vi "TiMicSDK.vi"() -> ()   [LabVIEW 2011]
uses:
  TILLPhotonics/DevID.ctl
panel:
  out "Value":string
  out "error out":errorcluster
  out "command":string
  # "version without z"
  # "*.z=\"1..\"\n*.x=\"...\"\n*.y=\"...\"\n*.f1=\"..\"\n*.turret=\"...\"\njeweils .set werte"
  # "stage.x.set=\"update\" for read"
  # "remember state! arrival time? not to sent new command before arrival!"
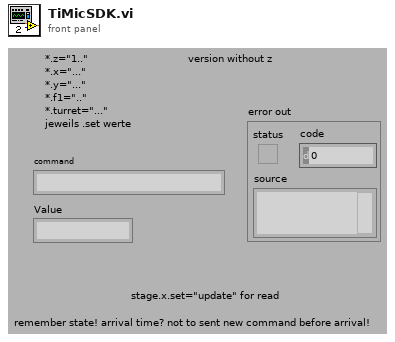
[diagram p1: front panel]
types:
  T1 = enum16{"None/#Datasets", "Clear", "TagValueOf#", "AddValues", "ReadValue", "ChangeValue", "Get all"}
  T2 = cluster{"default value 2":dbl, "default value 1":dbl}
  T3 = typedef "DevID.ctl" = i32
  T4 = enum16{"no error", "missing axis", "missing Z axis", "missing Filter", "iMic not initialized", "no property", "wrong handle", "protocol not finished", "user parameter to long (>32 bits)", "no user parameter handle", "failed to open comport", "failed to initialize"}
  T5 = cluster{bool, "output param":enum16{"no error", "missing axis", "missing Z axis", "missing Filter", "iMic not initialized", "no property", "wrong handle", "protocol not finished", "user parameter to long (>32 bits)", "no user parameter handle", "failed to open comport", "failed to initialize"}, string}
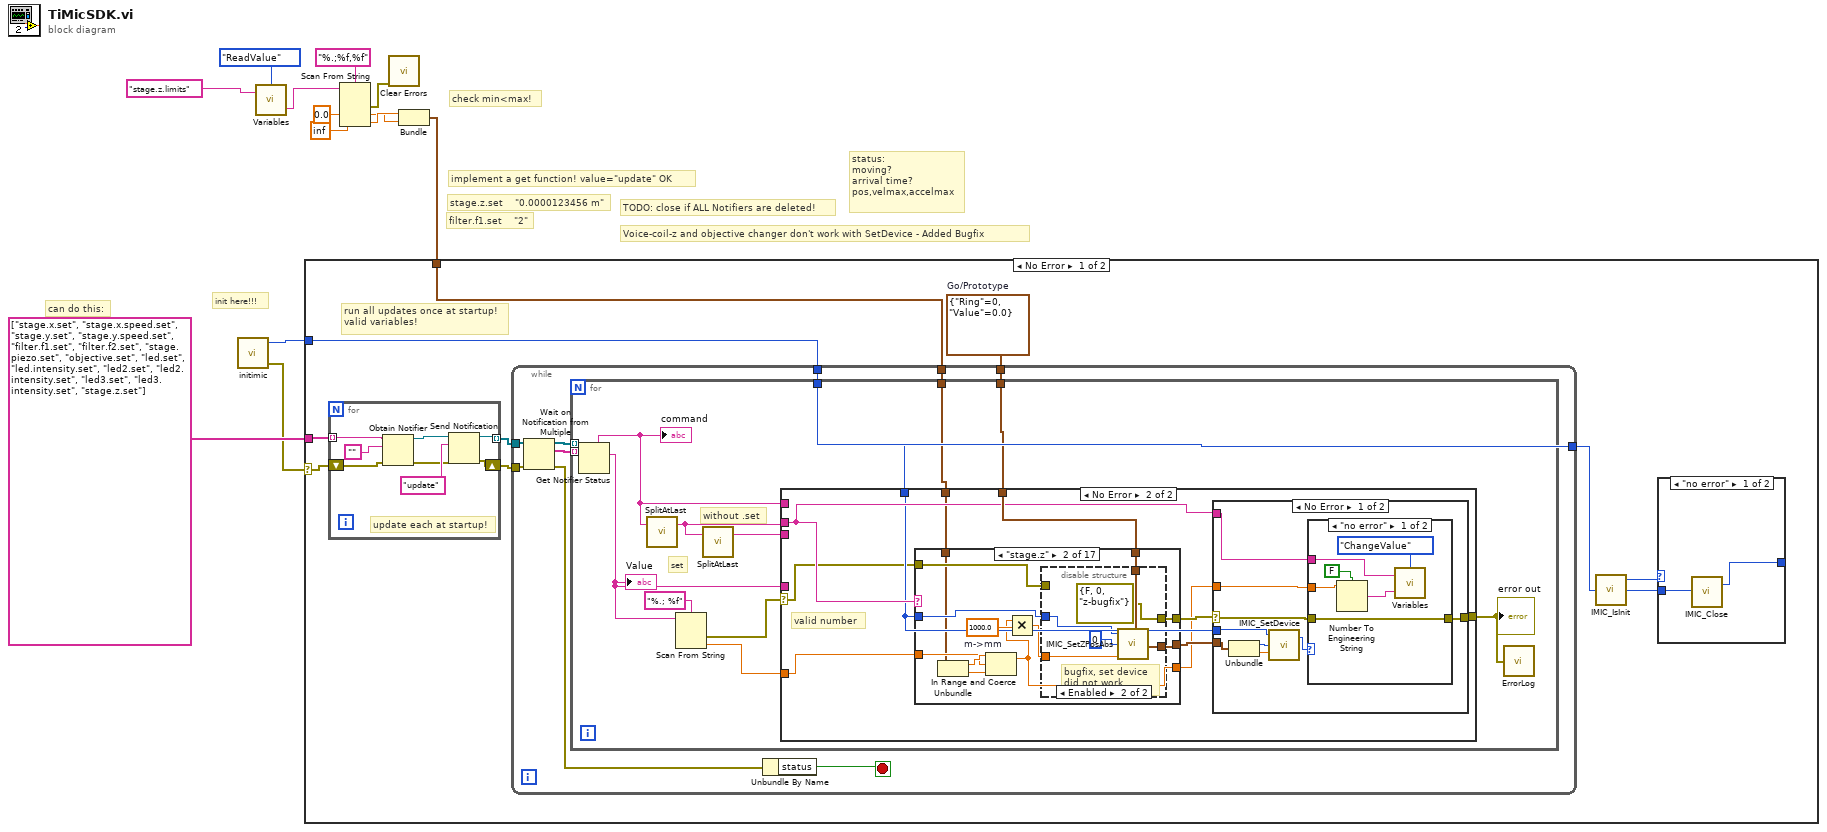
[diagram p0: block diagram]
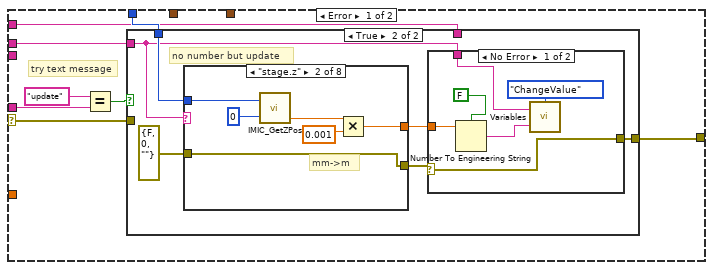
[diagram p3: hidden frame]
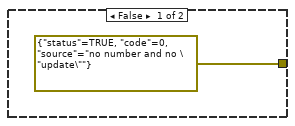
[diagram p4: hidden frame]
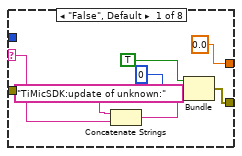
[diagram p6: hidden frame]
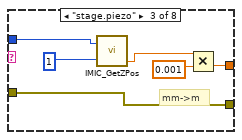
[diagram p7: hidden frame]
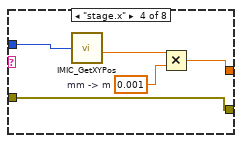
[diagram p8: hidden frame]
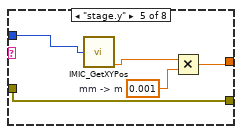
[diagram p9: hidden frame]
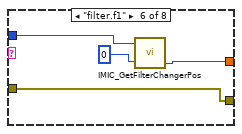
[diagram p10: hidden frame]
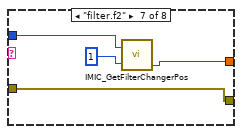
[diagram p11: hidden frame]
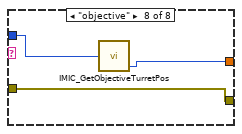
[diagram p12: hidden frame]
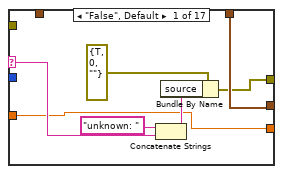
[diagram p13: hidden frame]
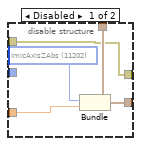
[diagram p14: hidden frame]
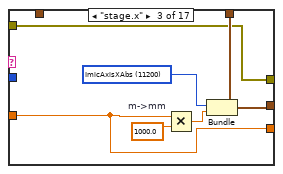
[diagram p15: hidden frame]
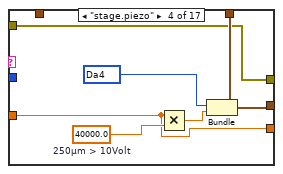
[diagram p16: hidden frame]
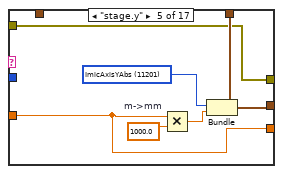
[diagram p17: hidden frame]
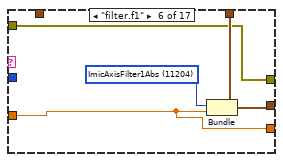
[diagram p18: hidden frame]
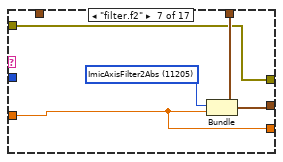
[diagram p19: hidden frame]
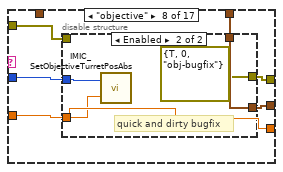
[diagram p20: hidden frame]
diagram:
  # "check min<max!"
  # "can do this:"
  # "Voice-coil-z and objective changer don't work with SetDevice - Added Bugfix"
  # "filter.f1.set    \"2\""
  # "status:\nmoving?\narrival time?\npos,velmax,accelmax"
  # "implement a get function! value=\"update\" OK"
  # "TODO: close if ALL Notifiers are deleted!"
  # "init here!!!"
  # "stage.z.set    \"0.0000123456 m\""
  n1 = call "initimic.vi"() -> ("handle"=w13:u64, "error out"=w11:errorcluster)  [unwired: 3 out]
  n2 = call "Variables.vi"("Tag in"="stage.z.limits", "Command"=T1."ReadValue") -> ("value out"=w8:string)  [unwired: 1 in, 2 out]
  n3 = Scan From String(format string="%.;%f,%f", input string=w8, default 1=0.0 ("default value 1"), default 2=inf ("default value 2")) -> (error out=w2:errorcluster, output 1=w3:dbl, output 2=w4:dbl)  [unwired: 2 in, 2 out]
  n4 = call <vilib>:"Clear Errors.vi"("error in (no error)"=w2) -> ()  [unwired: 7 out]
  n5 = Bundle("default value 2"=w4, "default value 1"=w3) -> (w1:T2)  [unwired: 1 out]
  n6 = case shown="No Error" w11 {
    selector: w11 -> [w15 _]
    tunnel: w13 -> [w23 _]
    tunnel: string[] ["stage.x.set", "stage.x.speed.set", "stage.y.set", "stage.y.speed.set", "filter.f1.set", "filter.f2.set", "stage.piezo.set", "objective.set", "led.set", "led.intensity.set", "led2.set", "led2.intensity.set", "led3.set", "led3.intensity.set", "stage.z.set"] -> [w18 _]
    tunnel: w1 -> [w14 _]
    frame No Error {
      w19 = cluster{"Ring":T3, "Value":dbl} {"Ring"=0, "Value"=0.0}  # Go/Prototype
      # "run all updates once at startup!\nvalid variables!"
      n7 = for {
        tunnel: w18 -> [w31] mode=indexing
        tunnel: [w25] -> w17 mode=indexing
        shift-right: [w24] -> w16
        shift-left: w15 -> [w29]
        # "update each at startup!"
        n8 = Obtain Notifier(name (unnamed)=w31, notification data type="", error in (no error)=w29) -> (notifier out=w27:refnum<notifier>, error out=w26:errorcluster)  [unwired: 1 in, 1 out]
        n9 = Send Notification(notification="update" ("Meldung"), notifier=w27, error in (no error)=w26) -> (notifier out=w25:refnum<notifier>, error out=w24:errorcluster)
      }
      n10 = while {
        tunnel: w17 -> [w38]
        tunnel: w23 -> [w42]
        tunnel: w16 -> [w40]
        tunnel: [w42] -> w21
        tunnel: w19 -> [w41]
        tunnel: w14 -> [w35]
        stop <- w43 stop-if-true
        n11 = Wait on Notification from Multiple(0:w38, 3:w40) -> (8:w37:refnum<notifier>[], 9:w36:string[], 11:w39:errorcluster)  [unwired: 3 out]
        n12 = for {
          tunnel: w42 -> [w55]
          tunnel: w41 -> [w54]
          tunnel: w37 -> [w53] mode=indexing
          tunnel: w36 -> [_] mode=indexing
          tunnel: w35 -> [w44]
          # "without .set"
          # "set"
          n13 = Get Notifier Status(notifier=w53) -> (notifier name=w52:string, current notification=w46:string)  [unwired: 1 in, 3 out]
          "command" <- w52
          "Value" <- w46
          n14 = call "SplitAtLast.vi"("In-String"=w52) -> ("Front (default)"=w51:string)  [unwired: 1 in, 1 out]
          n15 = Scan From String(format string="%.; %f", input string=w46) -> (error out=w47:errorcluster, output 1=w48:dbl)  [unwired: 2 in, 3 out]
          n16 = call "SplitAtLast.vi"("In-String"=w51) -> ("Front (default)"=w50:string)  [unwired: 1 in, 1 out]
          n17 = case shown="No Error" w47 {
            selector: w47 -> [w61 w119]
            tunnel: [w62 w127] -> w45
            tunnel: w55 -> [w63 w122]
            tunnel: w51 -> [w56 w123]
            tunnel: w52 -> [w60 _]
            tunnel: w54 -> [_ w126]
            tunnel: w50 -> [_ _]
            tunnel: w48 -> [_ w121]
            tunnel: w46 -> [w59 _]
            tunnel: w44 -> [_ w118]
            frame Error {
              # "try text message"
              n18 = Equal?(x="update", y=w59) -> (x = y?=w57:bool)
              n19 = case shown="True" w57 {
                tunnel: w63 -> [_ w70]
                tunnel: [errorcluster {"status"=TRUE, "code"=0, "source"="no number and no \"update\""} ("error out") w69] -> w62
                tunnel: w61 -> [_ _]
                tunnel: w60 -> [_ _]
                tunnel: w56 -> [_ w67]
                frame False {
                }
                frame True {
                  # "no number but update"
                  n20 = case shown="\"stage.z\"" w67 {
                    selector: w67 -> [w82 _ _ _ _ _ _ _]
                    tunnel: w70 -> [_ w90 w96 w101 w105 w110 w113 w117]
                    tunnel: [0.0 ("zpos") w86 w92 w98 w103 w108 w112 w116] -> w68
                    tunnel: errorcluster {"status"=FALSE, "code"=0, "source"=""} ("error out") -> [_ w85 w91 w97 w102 w107 w111 w115]
                    tunnel: [w81 w85 w91 w97 w102 w107 w111 w115] -> w65
                    frame "False", Default {
                      n21 = Concatenate Strings("TiMicSDK:update of unknown:" ("source"), w82) -> (w78:string)
                      n22 = Bundle("status"=TRUE, "code"=0, w78) -> (w81:cluster{"status":bool, "code":i32, string})  [unwired: 1 out]
                    }
                    frame "stage.z" {
                      # "mm->m"
                      n23 = call "IMIC_GetZPos.vi"("handle"=w90, "index"=0) -> ("zpos"=w87:dbl)  [unwired: 2 out]
                      n24 = Multiply(x=w87, y=0.001) -> (x*y=w86:dbl)
                    }
                    frame "stage.piezo" {
                      # "mm->m"
                      n25 = call "IMIC_GetZPos.vi"("handle"=w96, "index"=1) -> ("zpos"=w93:dbl)  [unwired: 2 out]
                      n26 = Multiply(x=w93, y=0.001) -> (x*y=w92:dbl)
                    }
                    frame "stage.x" {
                      w99 = 0.001  # mm -> m
                      n27 = call "IMIC_GetXYPos.vi"("handle"=w101) -> ("xpos"=w100:dbl)  [unwired: 3 out]
                      n28 = Multiply(x=w100, y=w99) -> (x*y=w98:dbl)
                    }
                    frame "stage.y" {
                      w106 = 0.001  # mm -> m
                      n29 = call "IMIC_GetXYPos.vi"("handle"=w105) -> ("ypos"=w104:dbl)  [unwired: 3 out]
                      n30 = Multiply(x=w104, y=w106) -> (x*y=w103:dbl)
                    }
                    frame "filter.f1" {
                      n31 = call "IMIC_GetFilterChangerPos.vi"("handle"=w110, "index"=0) -> ("Filter"=w108:i32)  [unwired: 2 out]
                    }
                    frame "filter.f2" {
                      n32 = call "IMIC_GetFilterChangerPos.vi"("handle"=w113, "index"=1) -> ("Filter"=w112:i32)  [unwired: 2 out]
                    }
                    frame "objective" {
                      n33 = call "IMIC_GetObjectiveTurretPos.vi"("handle"=w117) -> ("Objective"=w116:i32)  [unwired: 2 out]
                    }
                  }
                  n34 = case shown="No Error" w65 {
                    selector: w65 -> [w71 w77]
                    tunnel: [w71 w77] -> w69
                    tunnel: w68 -> [w73 _]
                    tunnel: w67 -> [w72 _]
                    frame No Error {
                      n35 = Number To Engineering String(1:FALSE ("use system decimal point (T)"), 4:w73) -> (0:w76:string)  [unwired: 2 out]
                      n36 = call "Variables.vi"("value"=w76, "Tag in"=w72, "Command"=T1."ChangeValue") -> ()  [unwired: 3 out]
                    }
                    frame Error {
                    }
                  }
                }
              }
            }
            frame No Error {
              # "valid number"
              n37 = case shown="\"stage.z\"" w123 {
                selector: w123 -> [w132 _ _ _ _ _ _ _ _ _ _ _ _ _ _ _ _]
                tunnel: w121 -> [w128 w137 w157 w164 w171 w178 w183 w190 w203 w213 w223 w237 w246 w254 w261 w269 w278]
                tunnel: [w129 w141 w159 w167 w173 w179 w184 w188 w205 w214 w224 w233 w242 w250 w257 w265 w274] -> w124
                tunnel: [w134 w144 w161 w169 w175 w181 w186 w193 w206 w216 w225 w240 w248 w256 w259 w267 w276] -> w125
                tunnel: w126 -> [w134 w145 w162 w170 w176 w182 w187 w191 w204 w215 w226 w239 w247 w255 w258 w266 w275]
                tunnel: w119 -> [_ w142 w159 w167 w173 w179 w184 w189 w205 w214 w224 w233 w242 w250 w257 w265 w274]
                tunnel: w122 -> [_ w140 _ _ _ _ _ w192 _ _ _ _ _ _ _ _ _]
                tunnel: [w128 w136 w157 w164 w171 w178 w183 w190 w203 w213 w223 w234 w243 w251 w260 w268 w277] -> w120
                tunnel: w118 -> [_ w135 _ _ _ _ _ _ _ _ _ _ _ _ _ _ _]
                frame "False", Default {
                  n38 = Concatenate Strings("unknown: ", w132) -> (w131:string)
                  n39 = Bundle By Name(cluster=errorcluster {"status"=TRUE, "code"=0, "source"=""} ("error out"), "source"=w131) -> (w129:errorcluster)
                }
                frame "stage.z" {
                  w146 = 1000.0  # m->mm
                  n40 = Unbundle(w135) -> ("default value 2"=w138:dbl, "default value 1"=w139:dbl)
                  n41 = In Range and Coerce(upper limit=w138, x=w137, lower limit=w139) -> (coerced(x)=w136:dbl)  [unwired: 1 out]
                  n42 = Multiply(x=w136, y=w146) -> (x*y=w143:dbl)
                  n43 = disable-structure shown="Enabled" {
                    disable-tunnel: w145 -> [w151 w156]
                    disable-tunnel: [w150 w156] -> w144
                    disable-tunnel: w143 -> [w148 w153]
                    disable-tunnel: w142 -> [w147 _]
                    disable-tunnel: [w147 errorcluster {"status"=FALSE, "code"=0, "source"="z-bugfix"} ("error in (no error)")] -> w141
                    disable-tunnel: w140 -> [_ w154]
                    frame Disabled {
                      w149 = 11202 items=["EndLoop"=-2, "Loop"=-1, "Invalid"=0, "TriggerPolyV"=1, "TriggerCamera"=2, "SyncCamera"=3, "Do1"=1000, "Do2"=1001, "Do3"=1002, "Do4"=1003, "Do5"=1004, "Do6"=1005, "Do7"=1006, "Do8"=1007, "Do9"=1008, "Do10"=1009, "Do11"=1010, "Do12"=1011, "Do13"=1012, "Do14"=1013, "Do15"=1014, "Do16"=1015, "Do17"=1016, "Do18"=1017, "Do19"=1018, "Do20"=1019, "Do21"=1020, "Do22"=1021, "Do23"=1022, "Do24"=1023, "Do_End"=1024, "Da1"=2000, "Da2"=2001, "Da3"=2002, "Da4"=2003, "Da5"=2004, "Da6"=2005, "Da7"=2006, "Da8"=2007, "DaIncr_First"=2008, "Da1Incr"=2100, "Da2Incr"=2101, "Da3Incr"=2102, "Da4Incr"=2103, "Da5Incr"=2104, "Da6Incr"=2105, "Da7Incr"=2106, "Da8Incr"=2107, "Da1Raw"=2200, "Da2Raw"=2201, "Da3Raw"=2202, "Da4Raw"=2203, "Da5Raw"=2204, "Da6Raw"=2205, "Da7Raw"=2206, "Da8Raw"=2207, "Da1RawIncr"=2300, "Da2RawIncr"=2301, "Da3RawIncr"=2302, "Da4RawIncr"=2303, "Da5RawIncr"=2304, "Da6RawIncr"=2305, "Da7RawIncr"=2306, "Da8RawIncr"=2307, "Uart1"=3000, "Uart2"=3001, "Uart3"=3002, "Uart_End"=3003, "Di1"=4000, "Di2"=4001, "Di3"=4002, "Di4"=4003, "Di5"=4004, "Di6"=4005, "Di7"=4006, "Di8"=4007, "Di9"=4008, "Di10"=4009, "Di11"=4010, "Di12"=4011, "Di13"=4012, "Di14"=4013, "Di15"=4014, "Di16"=4015, "Di17"=4016, "Di18"=4017, "Di19"=4018, "Di20"=4019, "Di21"=4020, "Di22"=4021, "Di23"=4022, "Di24"=4023, "Di_End"=4024, "ICU_End"=4025, "LedIllum"=10000, "ImicAxisXRel"=11000, "ImicAxisYRel"=11001, "ImicAxisZRel"=11002, "ImicAxisTurretRel"=11003, "ImicAxisFilter1Rel"=11004, "ImicAxisFilter2Rel"=11005, "ImicAxis_End"=11006, "ImicAxisXAbs"=11200, "ImicAxisYAbs"=11201, "ImicAxisZAbs"=11202, "ImicAxisTurretAbs"=11203, "ImicAxisFilter1Abs"=11204, "ImicAxisFilter2Abs"=11205, "ImicAxisXVel"=11300, "ImicAxisYVel"=11301, "ImicAxisZVel"=11302, "ImicAxisTurretVel"=11303, "ImicAxisFilter1Vel"=11304, "ImicAxisFilter2Vel"=11305, "ImicAxisXMoving"=11400, "ImicAxisYMoving"=11401, "ImicAxisZMoving"=11402, "ImicAxisTurretMoving"=11403, "ImicAxisFilter1Moving"=11404, "ImicAxisFilter2Moving"=11405, "ImicPiezoClip"=12001, "ImicPiezo"=12002, "IMIC_End"=12003] ("DeviceID")
                      n44 = Bundle(cluster=w151, "Ring"=w149, "Value"=w148) -> (w150:cluster{"Ring":T3, "Value":dbl})
                    }
                    frame Enabled {
                      # "bugfix, set device \ndid not work"
                      n45 = call "IMIC_SetZPosAbs.vi"("zpos"=w153, "index"=0, "handle"=w154) -> ()  [unwired: 2 out]
                    }
                  }
                }
                frame "stage.x" {
                  w160 = 11200 items=["EndLoop"=-2, "Loop"=-1, "Invalid"=0, "TriggerPolyV"=1, "TriggerCamera"=2, "SyncCamera"=3, "Do1"=1000, "Do2"=1001, "Do3"=1002, "Do4"=1003, "Do5"=1004, "Do6"=1005, "Do7"=1006, "Do8"=1007, "Do9"=1008, "Do10"=1009, "Do11"=1010, "Do12"=1011, "Do13"=1012, "Do14"=1013, "Do15"=1014, "Do16"=1015, "Do17"=1016, "Do18"=1017, "Do19"=1018, "Do20"=1019, "Do21"=1020, "Do22"=1021, "Do23"=1022, "Do24"=1023, "Do_End"=1024, "Da1"=2000, "Da2"=2001, "Da3"=2002, "Da4"=2003, "Da5"=2004, "Da6"=2005, "Da7"=2006, "Da8"=2007, "DaIncr_First"=2008, "Da1Incr"=2100, "Da2Incr"=2101, "Da3Incr"=2102, "Da4Incr"=2103, "Da5Incr"=2104, "Da6Incr"=2105, "Da7Incr"=2106, "Da8Incr"=2107, "Da1Raw"=2200, "Da2Raw"=2201, "Da3Raw"=2202, "Da4Raw"=2203, "Da5Raw"=2204, "Da6Raw"=2205, "Da7Raw"=2206, "Da8Raw"=2207, "Da1RawIncr"=2300, "Da2RawIncr"=2301, "Da3RawIncr"=2302, "Da4RawIncr"=2303, "Da5RawIncr"=2304, "Da6RawIncr"=2305, "Da7RawIncr"=2306, "Da8RawIncr"=2307, "Uart1"=3000, "Uart2"=3001, "Uart3"=3002, "Uart_End"=3003, "Di1"=4000, "Di2"=4001, "Di3"=4002, "Di4"=4003, "Di5"=4004, "Di6"=4005, "Di7"=4006, "Di8"=4007, "Di9"=4008, "Di10"=4009, "Di11"=4010, "Di12"=4011, "Di13"=4012, "Di14"=4013, "Di15"=4014, "Di16"=4015, "Di17"=4016, "Di18"=4017, "Di19"=4018, "Di20"=4019, "Di21"=4020, "Di22"=4021, "Di23"=4022, "Di24"=4023, "Di_End"=4024, "ICU_End"=4025, "LedIllum"=10000, "ImicAxisXRel"=11000, "ImicAxisYRel"=11001, "ImicAxisZRel"=11002, "ImicAxisTurretRel"=11003, "ImicAxisFilter1Rel"=11004, "ImicAxisFilter2Rel"=11005, "ImicAxis_End"=11006, "ImicAxisXAbs"=11200, "ImicAxisYAbs"=11201, "ImicAxisZAbs"=11202, "ImicAxisTurretAbs"=11203, "ImicAxisFilter1Abs"=11204, "ImicAxisFilter2Abs"=11205, "ImicAxisXVel"=11300, "ImicAxisYVel"=11301, "ImicAxisZVel"=11302, "ImicAxisTurretVel"=11303, "ImicAxisFilter1Vel"=11304, "ImicAxisFilter2Vel"=11305, "ImicAxisXMoving"=11400, "ImicAxisYMoving"=11401, "ImicAxisZMoving"=11402, "ImicAxisTurretMoving"=11403, "ImicAxisFilter1Moving"=11404, "ImicAxisFilter2Moving"=11405, "ImicPiezoClip"=12001, "ImicPiezo"=12002, "IMIC_End"=12003] ("DeviceID")
                  w163 = 1000.0  # m->mm
                  n46 = Multiply(x=w157, y=w163) -> (x*y=w158:dbl)
                  n47 = Bundle(cluster=w162, "Ring"=w160, "Value"=w158) -> (w161:cluster{"Ring":T3, "Value":dbl})
                }
                frame "stage.piezo" {
                  w165 = 40000.0  # 250µm > 10Volt
                  w168 = 2003 items=["EndLoop"=-2, "Loop"=-1, "Invalid"=0, "TriggerPolyV"=1, "TriggerCamera"=2, "SyncCamera"=3, "Do1"=1000, "Do2"=1001, "Do3"=1002, "Do4"=1003, "Do5"=1004, "Do6"=1005, "Do7"=1006, "Do8"=1007, "Do9"=1008, "Do10"=1009, "Do11"=1010, "Do12"=1011, "Do13"=1012, "Do14"=1013, "Do15"=1014, "Do16"=1015, "Do17"=1016, "Do18"=1017, "Do19"=1018, "Do20"=1019, "Do21"=1020, "Do22"=1021, "Do23"=1022, "Do24"=1023, "Do_End"=1024, "Da1"=2000, "Da2"=2001, "Da3"=2002, "Da4"=2003, "Da5"=2004, "Da6"=2005, "Da7"=2006, "Da8"=2007, "DaIncr_First"=2008, "Da1Incr"=2100, "Da2Incr"=2101, "Da3Incr"=2102, "Da4Incr"=2103, "Da5Incr"=2104, "Da6Incr"=2105, "Da7Incr"=2106, "Da8Incr"=2107, "Da1Raw"=2200, "Da2Raw"=2201, "Da3Raw"=2202, "Da4Raw"=2203, "Da5Raw"=2204, "Da6Raw"=2205, "Da7Raw"=2206, "Da8Raw"=2207, "Da1RawIncr"=2300, "Da2RawIncr"=2301, "Da3RawIncr"=2302, "Da4RawIncr"=2303, "Da5RawIncr"=2304, "Da6RawIncr"=2305, "Da7RawIncr"=2306, "Da8RawIncr"=2307, "Uart1"=3000, "Uart2"=3001, "Uart3"=3002, "Uart_End"=3003, "Di1"=4000, "Di2"=4001, "Di3"=4002, "Di4"=4003, "Di5"=4004, "Di6"=4005, "Di7"=4006, "Di8"=4007, "Di9"=4008, "Di10"=4009, "Di11"=4010, "Di12"=4011, "Di13"=4012, "Di14"=4013, "Di15"=4014, "Di16"=4015, "Di17"=4016, "Di18"=4017, "Di19"=4018, "Di20"=4019, "Di21"=4020, "Di22"=4021, "Di23"=4022, "Di24"=4023, "Di_End"=4024, "ICU_End"=4025, "LedIllum"=10000, "ImicAxisXRel"=11000, "ImicAxisYRel"=11001, "ImicAxisZRel"=11002, "ImicAxisTurretRel"=11003, "ImicAxisFilter1Rel"=11004, "ImicAxisFilter2Rel"=11005, "ImicAxis_End"=11006, "ImicAxisXAbs"=11200, "ImicAxisYAbs"=11201, "ImicAxisZAbs"=11202, "ImicAxisTurretAbs"=11203, "ImicAxisFilter1Abs"=11204, "ImicAxisFilter2Abs"=11205, "ImicAxisXVel"=11300, "ImicAxisYVel"=11301, "ImicAxisZVel"=11302, "ImicAxisTurretVel"=11303, "ImicAxisFilter1Vel"=11304, "ImicAxisFilter2Vel"=11305, "ImicAxisXMoving"=11400, "ImicAxisYMoving"=11401, "ImicAxisZMoving"=11402, "ImicAxisTurretMoving"=11403, "ImicAxisFilter1Moving"=11404, "ImicAxisFilter2Moving"=11405, "ImicPiezoClip"=12001, "ImicPiezo"=12002, "IMIC_End"=12003] ("DeviceID")
                  n48 = Multiply(x=w164, y=w165) -> (x*y=w166:dbl)
                  n49 = Bundle(cluster=w170, "Ring"=w168, "Value"=w166) -> (w169:cluster{"Ring":T3, "Value":dbl})
                }
                frame "stage.y" {
                  w174 = 11201 items=["EndLoop"=-2, "Loop"=-1, "Invalid"=0, "TriggerPolyV"=1, "TriggerCamera"=2, "SyncCamera"=3, "Do1"=1000, "Do2"=1001, "Do3"=1002, "Do4"=1003, "Do5"=1004, "Do6"=1005, "Do7"=1006, "Do8"=1007, "Do9"=1008, "Do10"=1009, "Do11"=1010, "Do12"=1011, "Do13"=1012, "Do14"=1013, "Do15"=1014, "Do16"=1015, "Do17"=1016, "Do18"=1017, "Do19"=1018, "Do20"=1019, "Do21"=1020, "Do22"=1021, "Do23"=1022, "Do24"=1023, "Do_End"=1024, "Da1"=2000, "Da2"=2001, "Da3"=2002, "Da4"=2003, "Da5"=2004, "Da6"=2005, "Da7"=2006, "Da8"=2007, "DaIncr_First"=2008, "Da1Incr"=2100, "Da2Incr"=2101, "Da3Incr"=2102, "Da4Incr"=2103, "Da5Incr"=2104, "Da6Incr"=2105, "Da7Incr"=2106, "Da8Incr"=2107, "Da1Raw"=2200, "Da2Raw"=2201, "Da3Raw"=2202, "Da4Raw"=2203, "Da5Raw"=2204, "Da6Raw"=2205, "Da7Raw"=2206, "Da8Raw"=2207, "Da1RawIncr"=2300, "Da2RawIncr"=2301, "Da3RawIncr"=2302, "Da4RawIncr"=2303, "Da5RawIncr"=2304, "Da6RawIncr"=2305, "Da7RawIncr"=2306, "Da8RawIncr"=2307, "Uart1"=3000, "Uart2"=3001, "Uart3"=3002, "Uart_End"=3003, "Di1"=4000, "Di2"=4001, "Di3"=4002, "Di4"=4003, "Di5"=4004, "Di6"=4005, "Di7"=4006, "Di8"=4007, "Di9"=4008, "Di10"=4009, "Di11"=4010, "Di12"=4011, "Di13"=4012, "Di14"=4013, "Di15"=4014, "Di16"=4015, "Di17"=4016, "Di18"=4017, "Di19"=4018, "Di20"=4019, "Di21"=4020, "Di22"=4021, "Di23"=4022, "Di24"=4023, "Di_End"=4024, "ICU_End"=4025, "LedIllum"=10000, "ImicAxisXRel"=11000, "ImicAxisYRel"=11001, "ImicAxisZRel"=11002, "ImicAxisTurretRel"=11003, "ImicAxisFilter1Rel"=11004, "ImicAxisFilter2Rel"=11005, "ImicAxis_End"=11006, "ImicAxisXAbs"=11200, "ImicAxisYAbs"=11201, "ImicAxisZAbs"=11202, "ImicAxisTurretAbs"=11203, "ImicAxisFilter1Abs"=11204, "ImicAxisFilter2Abs"=11205, "ImicAxisXVel"=11300, "ImicAxisYVel"=11301, "ImicAxisZVel"=11302, "ImicAxisTurretVel"=11303, "ImicAxisFilter1Vel"=11304, "ImicAxisFilter2Vel"=11305, "ImicAxisXMoving"=11400, "ImicAxisYMoving"=11401, "ImicAxisZMoving"=11402, "ImicAxisTurretMoving"=11403, "ImicAxisFilter1Moving"=11404, "ImicAxisFilter2Moving"=11405, "ImicPiezoClip"=12001, "ImicPiezo"=12002, "IMIC_End"=12003] ("DeviceID")
                  w177 = 1000.0  # m->mm
                  n50 = Multiply(x=w171, y=w177) -> (x*y=w172:dbl)
                  n51 = Bundle(cluster=w176, "Ring"=w174, "Value"=w172) -> (w175:cluster{"Ring":T3, "Value":dbl})
                }
                frame "filter.f1" {
                  w180 = 11204 items=["EndLoop"=-2, "Loop"=-1, "Invalid"=0, "TriggerPolyV"=1, "TriggerCamera"=2, "SyncCamera"=3, "Do1"=1000, "Do2"=1001, "Do3"=1002, "Do4"=1003, "Do5"=1004, "Do6"=1005, "Do7"=1006, "Do8"=1007, "Do9"=1008, "Do10"=1009, "Do11"=1010, "Do12"=1011, "Do13"=1012, "Do14"=1013, "Do15"=1014, "Do16"=1015, "Do17"=1016, "Do18"=1017, "Do19"=1018, "Do20"=1019, "Do21"=1020, "Do22"=1021, "Do23"=1022, "Do24"=1023, "Do_End"=1024, "Da1"=2000, "Da2"=2001, "Da3"=2002, "Da4"=2003, "Da5"=2004, "Da6"=2005, "Da7"=2006, "Da8"=2007, "DaIncr_First"=2008, "Da1Incr"=2100, "Da2Incr"=2101, "Da3Incr"=2102, "Da4Incr"=2103, "Da5Incr"=2104, "Da6Incr"=2105, "Da7Incr"=2106, "Da8Incr"=2107, "Da1Raw"=2200, "Da2Raw"=2201, "Da3Raw"=2202, "Da4Raw"=2203, "Da5Raw"=2204, "Da6Raw"=2205, "Da7Raw"=2206, "Da8Raw"=2207, "Da1RawIncr"=2300, "Da2RawIncr"=2301, "Da3RawIncr"=2302, "Da4RawIncr"=2303, "Da5RawIncr"=2304, "Da6RawIncr"=2305, "Da7RawIncr"=2306, "Da8RawIncr"=2307, "Uart1"=3000, "Uart2"=3001, "Uart3"=3002, "Uart_End"=3003, "Di1"=4000, "Di2"=4001, "Di3"=4002, "Di4"=4003, "Di5"=4004, "Di6"=4005, "Di7"=4006, "Di8"=4007, "Di9"=4008, "Di10"=4009, "Di11"=4010, "Di12"=4011, "Di13"=4012, "Di14"=4013, "Di15"=4014, "Di16"=4015, "Di17"=4016, "Di18"=4017, "Di19"=4018, "Di20"=4019, "Di21"=4020, "Di22"=4021, "Di23"=4022, "Di24"=4023, "Di_End"=4024, "ICU_End"=4025, "LedIllum"=10000, "ImicAxisXRel"=11000, "ImicAxisYRel"=11001, "ImicAxisZRel"=11002, "ImicAxisTurretRel"=11003, "ImicAxisFilter1Rel"=11004, "ImicAxisFilter2Rel"=11005, "ImicAxis_End"=11006, "ImicAxisXAbs"=11200, "ImicAxisYAbs"=11201, "ImicAxisZAbs"=11202, "ImicAxisTurretAbs"=11203, "ImicAxisFilter1Abs"=11204, "ImicAxisFilter2Abs"=11205, "ImicAxisXVel"=11300, "ImicAxisYVel"=11301, "ImicAxisZVel"=11302, "ImicAxisTurretVel"=11303, "ImicAxisFilter1Vel"=11304, "ImicAxisFilter2Vel"=11305, "ImicAxisXMoving"=11400, "ImicAxisYMoving"=11401, "ImicAxisZMoving"=11402, "ImicAxisTurretMoving"=11403, "ImicAxisFilter1Moving"=11404, "ImicAxisFilter2Moving"=11405, "ImicPiezoClip"=12001, "ImicPiezo"=12002, "IMIC_End"=12003] ("DeviceID")
                  n52 = Bundle(cluster=w182, "Ring"=w180, "Value"=w178) -> (w181:cluster{"Ring":T3, "Value":dbl})
                }
                frame "filter.f2" {
                  w185 = 11205 items=["EndLoop"=-2, "Loop"=-1, "Invalid"=0, "TriggerPolyV"=1, "TriggerCamera"=2, "SyncCamera"=3, "Do1"=1000, "Do2"=1001, "Do3"=1002, "Do4"=1003, "Do5"=1004, "Do6"=1005, "Do7"=1006, "Do8"=1007, "Do9"=1008, "Do10"=1009, "Do11"=1010, "Do12"=1011, "Do13"=1012, "Do14"=1013, "Do15"=1014, "Do16"=1015, "Do17"=1016, "Do18"=1017, "Do19"=1018, "Do20"=1019, "Do21"=1020, "Do22"=1021, "Do23"=1022, "Do24"=1023, "Do_End"=1024, "Da1"=2000, "Da2"=2001, "Da3"=2002, "Da4"=2003, "Da5"=2004, "Da6"=2005, "Da7"=2006, "Da8"=2007, "DaIncr_First"=2008, "Da1Incr"=2100, "Da2Incr"=2101, "Da3Incr"=2102, "Da4Incr"=2103, "Da5Incr"=2104, "Da6Incr"=2105, "Da7Incr"=2106, "Da8Incr"=2107, "Da1Raw"=2200, "Da2Raw"=2201, "Da3Raw"=2202, "Da4Raw"=2203, "Da5Raw"=2204, "Da6Raw"=2205, "Da7Raw"=2206, "Da8Raw"=2207, "Da1RawIncr"=2300, "Da2RawIncr"=2301, "Da3RawIncr"=2302, "Da4RawIncr"=2303, "Da5RawIncr"=2304, "Da6RawIncr"=2305, "Da7RawIncr"=2306, "Da8RawIncr"=2307, "Uart1"=3000, "Uart2"=3001, "Uart3"=3002, "Uart_End"=3003, "Di1"=4000, "Di2"=4001, "Di3"=4002, "Di4"=4003, "Di5"=4004, "Di6"=4005, "Di7"=4006, "Di8"=4007, "Di9"=4008, "Di10"=4009, "Di11"=4010, "Di12"=4011, "Di13"=4012, "Di14"=4013, "Di15"=4014, "Di16"=4015, "Di17"=4016, "Di18"=4017, "Di19"=4018, "Di20"=4019, "Di21"=4020, "Di22"=4021, "Di23"=4022, "Di24"=4023, "Di_End"=4024, "ICU_End"=4025, "LedIllum"=10000, "ImicAxisXRel"=11000, "ImicAxisYRel"=11001, "ImicAxisZRel"=11002, "ImicAxisTurretRel"=11003, "ImicAxisFilter1Rel"=11004, "ImicAxisFilter2Rel"=11005, "ImicAxis_End"=11006, "ImicAxisXAbs"=11200, "ImicAxisYAbs"=11201, "ImicAxisZAbs"=11202, "ImicAxisTurretAbs"=11203, "ImicAxisFilter1Abs"=11204, "ImicAxisFilter2Abs"=11205, "ImicAxisXVel"=11300, "ImicAxisYVel"=11301, "ImicAxisZVel"=11302, "ImicAxisTurretVel"=11303, "ImicAxisFilter1Vel"=11304, "ImicAxisFilter2Vel"=11305, "ImicAxisXMoving"=11400, "ImicAxisYMoving"=11401, "ImicAxisZMoving"=11402, "ImicAxisTurretMoving"=11403, "ImicAxisFilter1Moving"=11404, "ImicAxisFilter2Moving"=11405, "ImicPiezoClip"=12001, "ImicPiezo"=12002, "IMIC_End"=12003] ("DeviceID")
                  n53 = Bundle(cluster=w187, "Ring"=w185, "Value"=w183) -> (w186:cluster{"Ring":T3, "Value":dbl})
                }
                frame "objective" {
                  n54 = disable-structure shown="Enabled" {
                    disable-tunnel: [w197 w200] -> w193
                    disable-tunnel: w192 -> [_ w202]
                    disable-tunnel: w191 -> [w196 w200]
                    disable-tunnel: w190 -> [w195 w201]
                    disable-tunnel: w189 -> [w194 _]
                    disable-tunnel: [w194 errorcluster {"status"=TRUE, "code"=0, "source"="obj-bugfix"} ("error in (no error)")] -> w188
                    frame Disabled {
                      w198 = 11203 items=["EndLoop"=-2, "Loop"=-1, "Invalid"=0, "TriggerPolyV"=1, "TriggerCamera"=2, "SyncCamera"=3, "Do1"=1000, "Do2"=1001, "Do3"=1002, "Do4"=1003, "Do5"=1004, "Do6"=1005, "Do7"=1006, "Do8"=1007, "Do9"=1008, "Do10"=1009, "Do11"=1010, "Do12"=1011, "Do13"=1012, "Do14"=1013, "Do15"=1014, "Do16"=1015, "Do17"=1016, "Do18"=1017, "Do19"=1018, "Do20"=1019, "Do21"=1020, "Do22"=1021, "Do23"=1022, "Do24"=1023, "Do_End"=1024, "Da1"=2000, "Da2"=2001, "Da3"=2002, "Da4"=2003, "Da5"=2004, "Da6"=2005, "Da7"=2006, "Da8"=2007, "DaIncr_First"=2008, "Da1Incr"=2100, "Da2Incr"=2101, "Da3Incr"=2102, "Da4Incr"=2103, "Da5Incr"=2104, "Da6Incr"=2105, "Da7Incr"=2106, "Da8Incr"=2107, "Da1Raw"=2200, "Da2Raw"=2201, "Da3Raw"=2202, "Da4Raw"=2203, "Da5Raw"=2204, "Da6Raw"=2205, "Da7Raw"=2206, "Da8Raw"=2207, "Da1RawIncr"=2300, "Da2RawIncr"=2301, "Da3RawIncr"=2302, "Da4RawIncr"=2303, "Da5RawIncr"=2304, "Da6RawIncr"=2305, "Da7RawIncr"=2306, "Da8RawIncr"=2307, "Uart1"=3000, "Uart2"=3001, "Uart3"=3002, "Uart_End"=3003, "Di1"=4000, "Di2"=4001, "Di3"=4002, "Di4"=4003, "Di5"=4004, "Di6"=4005, "Di7"=4006, "Di8"=4007, "Di9"=4008, "Di10"=4009, "Di11"=4010, "Di12"=4011, "Di13"=4012, "Di14"=4013, "Di15"=4014, "Di16"=4015, "Di17"=4016, "Di18"=4017, "Di19"=4018, "Di20"=4019, "Di21"=4020, "Di22"=4021, "Di23"=4022, "Di24"=4023, "Di_End"=4024, "ICU_End"=4025, "LedIllum"=10000, "ImicAxisXRel"=11000, "ImicAxisYRel"=11001, "ImicAxisZRel"=11002, "ImicAxisTurretRel"=11003, "ImicAxisFilter1Rel"=11004, "ImicAxisFilter2Rel"=11005, "ImicAxis_End"=11006, "ImicAxisXAbs"=11200, "ImicAxisYAbs"=11201, "ImicAxisZAbs"=11202, "ImicAxisTurretAbs"=11203, "ImicAxisFilter1Abs"=11204, "ImicAxisFilter2Abs"=11205, "ImicAxisXVel"=11300, "ImicAxisYVel"=11301, "ImicAxisZVel"=11302, "ImicAxisTurretVel"=11303, "ImicAxisFilter1Vel"=11304, "ImicAxisFilter2Vel"=11305, "ImicAxisXMoving"=11400, "ImicAxisYMoving"=11401, "ImicAxisZMoving"=11402, "ImicAxisTurretMoving"=11403, "ImicAxisFilter1Moving"=11404, "ImicAxisFilter2Moving"=11405, "ImicPiezoClip"=12001, "ImicPiezo"=12002, "IMIC_End"=12003] ("DeviceID")
                      n55 = Bundle(cluster=w196, "Ring"=w198, "Value"=w195) -> (w197:cluster{"Ring":T3, "Value":dbl})
                    }
                    frame Enabled {
                      # "quick and dirty bugfix"
                      n56 = call "IMIC_SetObjectiveTurretPosAbs.vi"("ObjectivePosAbs"=w201, "handle"=w202) -> ()  [unwired: 2 out]
                    }
                  }
                }
                frame "stage.z.speed" {
                  w212 = 1000.0  # m->mm
                  w211 = 11302 items=["EndLoop"=-2, "Loop"=-1, "Invalid"=0, "TriggerPolyV"=1, "TriggerCamera"=2, "SyncCamera"=3, "Do1"=1000, "Do2"=1001, "Do3"=1002, "Do4"=1003, "Do5"=1004, "Do6"=1005, "Do7"=1006, "Do8"=1007, "Do9"=1008, "Do10"=1009, "Do11"=1010, "Do12"=1011, "Do13"=1012, "Do14"=1013, "Do15"=1014, "Do16"=1015, "Do17"=1016, "Do18"=1017, "Do19"=1018, "Do20"=1019, "Do21"=1020, "Do22"=1021, "Do23"=1022, "Do24"=1023, "Do_End"=1024, "Da1"=2000, "Da2"=2001, "Da3"=2002, "Da4"=2003, "Da5"=2004, "Da6"=2005, "Da7"=2006, "Da8"=2007, "DaIncr_First"=2008, "Da1Incr"=2100, "Da2Incr"=2101, "Da3Incr"=2102, "Da4Incr"=2103, "Da5Incr"=2104, "Da6Incr"=2105, "Da7Incr"=2106, "Da8Incr"=2107, "Da1Raw"=2200, "Da2Raw"=2201, "Da3Raw"=2202, "Da4Raw"=2203, "Da5Raw"=2204, "Da6Raw"=2205, "Da7Raw"=2206, "Da8Raw"=2207, "Da1RawIncr"=2300, "Da2RawIncr"=2301, "Da3RawIncr"=2302, "Da4RawIncr"=2303, "Da5RawIncr"=2304, "Da6RawIncr"=2305, "Da7RawIncr"=2306, "Da8RawIncr"=2307, "Uart1"=3000, "Uart2"=3001, "Uart3"=3002, "Uart_End"=3003, "Di1"=4000, "Di2"=4001, "Di3"=4002, "Di4"=4003, "Di5"=4004, "Di6"=4005, "Di7"=4006, "Di8"=4007, "Di9"=4008, "Di10"=4009, "Di11"=4010, "Di12"=4011, "Di13"=4012, "Di14"=4013, "Di15"=4014, "Di16"=4015, "Di17"=4016, "Di18"=4017, "Di19"=4018, "Di20"=4019, "Di21"=4020, "Di22"=4021, "Di23"=4022, "Di24"=4023, "Di_End"=4024, "ICU_End"=4025, "LedIllum"=10000, "ImicAxisXRel"=11000, "ImicAxisYRel"=11001, "ImicAxisZRel"=11002, "ImicAxisTurretRel"=11003, "ImicAxisFilter1Rel"=11004, "ImicAxisFilter2Rel"=11005, "ImicAxis_End"=11006, "ImicAxisXAbs"=11200, "ImicAxisYAbs"=11201, "ImicAxisZAbs"=11202, "ImicAxisTurretAbs"=11203, "ImicAxisFilter1Abs"=11204, "ImicAxisFilter2Abs"=11205, "ImicAxisXVel"=11300, "ImicAxisYVel"=11301, "ImicAxisZVel"=11302, "ImicAxisTurretVel"=11303, "ImicAxisFilter1Vel"=11304, "ImicAxisFilter2Vel"=11305, "ImicAxisXMoving"=11400, "ImicAxisYMoving"=11401, "ImicAxisZMoving"=11402, "ImicAxisTurretMoving"=11403, "ImicAxisFilter1Moving"=11404, "ImicAxisFilter2Moving"=11405, "ImicPiezoClip"=12001, "ImicPiezo"=12002, "IMIC_End"=12003] ("DeviceID")
                  n57 = Not Equal To 0?(x=w203) -> (x != 0?=w208:bool)
                  n58 = Select(t=w203, s=w208, f=0.001) -> (s? t:f=w207:dbl)
                  n59 = Multiply(x=w207, y=w212) -> (x*y=w210:dbl)
                  n60 = Bundle(cluster=w204, "Ring"=w211, "Value"=w210) -> (w206:cluster{"Ring":T3, "Value":dbl})
                }
                frame "stage.x.speed" {
                  w222 = 1000.0  # m->mm
                  w221 = 11300 items=["EndLoop"=-2, "Loop"=-1, "Invalid"=0, "TriggerPolyV"=1, "TriggerCamera"=2, "SyncCamera"=3, "Do1"=1000, "Do2"=1001, "Do3"=1002, "Do4"=1003, "Do5"=1004, "Do6"=1005, "Do7"=1006, "Do8"=1007, "Do9"=1008, "Do10"=1009, "Do11"=1010, "Do12"=1011, "Do13"=1012, "Do14"=1013, "Do15"=1014, "Do16"=1015, "Do17"=1016, "Do18"=1017, "Do19"=1018, "Do20"=1019, "Do21"=1020, "Do22"=1021, "Do23"=1022, "Do24"=1023, "Do_End"=1024, "Da1"=2000, "Da2"=2001, "Da3"=2002, "Da4"=2003, "Da5"=2004, "Da6"=2005, "Da7"=2006, "Da8"=2007, "DaIncr_First"=2008, "Da1Incr"=2100, "Da2Incr"=2101, "Da3Incr"=2102, "Da4Incr"=2103, "Da5Incr"=2104, "Da6Incr"=2105, "Da7Incr"=2106, "Da8Incr"=2107, "Da1Raw"=2200, "Da2Raw"=2201, "Da3Raw"=2202, "Da4Raw"=2203, "Da5Raw"=2204, "Da6Raw"=2205, "Da7Raw"=2206, "Da8Raw"=2207, "Da1RawIncr"=2300, "Da2RawIncr"=2301, "Da3RawIncr"=2302, "Da4RawIncr"=2303, "Da5RawIncr"=2304, "Da6RawIncr"=2305, "Da7RawIncr"=2306, "Da8RawIncr"=2307, "Uart1"=3000, "Uart2"=3001, "Uart3"=3002, "Uart_End"=3003, "Di1"=4000, "Di2"=4001, "Di3"=4002, "Di4"=4003, "Di5"=4004, "Di6"=4005, "Di7"=4006, "Di8"=4007, "Di9"=4008, "Di10"=4009, "Di11"=4010, "Di12"=4011, "Di13"=4012, "Di14"=4013, "Di15"=4014, "Di16"=4015, "Di17"=4016, "Di18"=4017, "Di19"=4018, "Di20"=4019, "Di21"=4020, "Di22"=4021, "Di23"=4022, "Di24"=4023, "Di_End"=4024, "ICU_End"=4025, "LedIllum"=10000, "ImicAxisXRel"=11000, "ImicAxisYRel"=11001, "ImicAxisZRel"=11002, "ImicAxisTurretRel"=11003, "ImicAxisFilter1Rel"=11004, "ImicAxisFilter2Rel"=11005, "ImicAxis_End"=11006, "ImicAxisXAbs"=11200, "ImicAxisYAbs"=11201, "ImicAxisZAbs"=11202, "ImicAxisTurretAbs"=11203, "ImicAxisFilter1Abs"=11204, "ImicAxisFilter2Abs"=11205, "ImicAxisXVel"=11300, "ImicAxisYVel"=11301, "ImicAxisZVel"=11302, "ImicAxisTurretVel"=11303, "ImicAxisFilter1Vel"=11304, "ImicAxisFilter2Vel"=11305, "ImicAxisXMoving"=11400, "ImicAxisYMoving"=11401, "ImicAxisZMoving"=11402, "ImicAxisTurretMoving"=11403, "ImicAxisFilter1Moving"=11404, "ImicAxisFilter2Moving"=11405, "ImicPiezoClip"=12001, "ImicPiezo"=12002, "IMIC_End"=12003] ("DeviceID")
                  n61 = Not Equal To 0?(x=w213) -> (x != 0?=w218:bool)
                  n62 = Select(t=w213, s=w218, f=0.02) -> (s? t:f=w217:dbl)
                  n63 = Multiply(x=w217, y=w222) -> (x*y=w220:dbl)
                  n64 = Bundle(cluster=w215, "Ring"=w221, "Value"=w220) -> (w216:cluster{"Ring":T3, "Value":dbl})
                }
                frame "stage.y.speed" {
                  w232 = 1000.0  # m->mm
                  w231 = 11301 items=["EndLoop"=-2, "Loop"=-1, "Invalid"=0, "TriggerPolyV"=1, "TriggerCamera"=2, "SyncCamera"=3, "Do1"=1000, "Do2"=1001, "Do3"=1002, "Do4"=1003, "Do5"=1004, "Do6"=1005, "Do7"=1006, "Do8"=1007, "Do9"=1008, "Do10"=1009, "Do11"=1010, "Do12"=1011, "Do13"=1012, "Do14"=1013, "Do15"=1014, "Do16"=1015, "Do17"=1016, "Do18"=1017, "Do19"=1018, "Do20"=1019, "Do21"=1020, "Do22"=1021, "Do23"=1022, "Do24"=1023, "Do_End"=1024, "Da1"=2000, "Da2"=2001, "Da3"=2002, "Da4"=2003, "Da5"=2004, "Da6"=2005, "Da7"=2006, "Da8"=2007, "DaIncr_First"=2008, "Da1Incr"=2100, "Da2Incr"=2101, "Da3Incr"=2102, "Da4Incr"=2103, "Da5Incr"=2104, "Da6Incr"=2105, "Da7Incr"=2106, "Da8Incr"=2107, "Da1Raw"=2200, "Da2Raw"=2201, "Da3Raw"=2202, "Da4Raw"=2203, "Da5Raw"=2204, "Da6Raw"=2205, "Da7Raw"=2206, "Da8Raw"=2207, "Da1RawIncr"=2300, "Da2RawIncr"=2301, "Da3RawIncr"=2302, "Da4RawIncr"=2303, "Da5RawIncr"=2304, "Da6RawIncr"=2305, "Da7RawIncr"=2306, "Da8RawIncr"=2307, "Uart1"=3000, "Uart2"=3001, "Uart3"=3002, "Uart_End"=3003, "Di1"=4000, "Di2"=4001, "Di3"=4002, "Di4"=4003, "Di5"=4004, "Di6"=4005, "Di7"=4006, "Di8"=4007, "Di9"=4008, "Di10"=4009, "Di11"=4010, "Di12"=4011, "Di13"=4012, "Di14"=4013, "Di15"=4014, "Di16"=4015, "Di17"=4016, "Di18"=4017, "Di19"=4018, "Di20"=4019, "Di21"=4020, "Di22"=4021, "Di23"=4022, "Di24"=4023, "Di_End"=4024, "ICU_End"=4025, "LedIllum"=10000, "ImicAxisXRel"=11000, "ImicAxisYRel"=11001, "ImicAxisZRel"=11002, "ImicAxisTurretRel"=11003, "ImicAxisFilter1Rel"=11004, "ImicAxisFilter2Rel"=11005, "ImicAxis_End"=11006, "ImicAxisXAbs"=11200, "ImicAxisYAbs"=11201, "ImicAxisZAbs"=11202, "ImicAxisTurretAbs"=11203, "ImicAxisFilter1Abs"=11204, "ImicAxisFilter2Abs"=11205, "ImicAxisXVel"=11300, "ImicAxisYVel"=11301, "ImicAxisZVel"=11302, "ImicAxisTurretVel"=11303, "ImicAxisFilter1Vel"=11304, "ImicAxisFilter2Vel"=11305, "ImicAxisXMoving"=11400, "ImicAxisYMoving"=11401, "ImicAxisZMoving"=11402, "ImicAxisTurretMoving"=11403, "ImicAxisFilter1Moving"=11404, "ImicAxisFilter2Moving"=11405, "ImicPiezoClip"=12001, "ImicPiezo"=12002, "IMIC_End"=12003] ("DeviceID")
                  n65 = Not Equal To 0?(x=w223) -> (x != 0?=w228:bool)
                  n66 = Select(t=w223, s=w228, f=0.02) -> (s? t:f=w229:dbl)
                  n67 = Multiply(x=w229, y=w232) -> (x*y=w230:dbl)
                  n68 = Bundle(cluster=w226, "Ring"=w231, "Value"=w230) -> (w225:cluster{"Ring":T3, "Value":dbl})
                }
                frame "led" {
                  w238 = 1025 items=["EndLoop"=-2, "Loop"=-1, "Invalid"=0, "TriggerPolyV"=1, "TriggerCamera"=2, "SyncCamera"=3, "Do1"=1000, "Do2"=1001, "Do3"=1002, "Do4"=1003, "Do5"=1004, "Do6"=1005, "Do7"=1006, "Do8"=1007, "Do9"=1008, "Do10"=1009, "Do11"=1010, "Do12"=1011, "Do13"=1012, "Do14"=1013, "Do15"=1014, "Do16"=1015, "Do17"=1016, "Do18"=1017, "Do19"=1018, "Do20"=1019, "Do21"=1020, "Do22"=1021, "Do23"=1022, "Do24"=1023, "Do25"=1024, "Do26"=1025, "Da1"=2000, "Da2"=2001, "Da3"=2002, "Da4"=2003, "Da5"=2004, "Da6"=2005, "Da7"=2006, "Da8"=2007, "DaIncr_First"=2008, "Da1Incr"=2100, "Da2Incr"=2101, "Da3Incr"=2102, "Da4Incr"=2103, "Da5Incr"=2104, "Da6Incr"=2105, "Da7Incr"=2106, "Da8Incr"=2107, "Da1Raw"=2200, "Da2Raw"=2201, "Da3Raw"=2202, "Da4Raw"=2203, "Da5Raw"=2204, "Da6Raw"=2205, "Da7Raw"=2206, "Da8Raw"=2207, "Da1RawIncr"=2300, "Da2RawIncr"=2301, "Da3RawIncr"=2302, "Da4RawIncr"=2303, "Da5RawIncr"=2304, "Da6RawIncr"=2305, "Da7RawIncr"=2306, "Da8RawIncr"=2307, "Uart1"=3000, "Uart2"=3001, "Uart3"=3002, "Uart_End"=3003, "Di1"=4000, "Di2"=4001, "Di3"=4002, "Di4"=4003, "Di5"=4004, "Di6"=4005, "Di7"=4006, "Di8"=4007, "Di9"=4008, "Di10"=4009, "Di11"=4010, "Di12"=4011, "Di13"=4012, "Di14"=4013, "Di15"=4014, "Di16"=4015, "Di17"=4016, "Di18"=4017, "Di19"=4018, "Di20"=4019, "Di21"=4020, "Di22"=4021, "Di23"=4022, "Di24"=4023, "Di_End"=4024, "ICU_End"=4025, "LedIllum"=10000, "ImicAxisXRel"=11000, "ImicAxisYRel"=11001, "ImicAxisZRel"=11002, "ImicAxisTurretRel"=11003, "ImicAxisFilter1Rel"=11004, "ImicAxisFilter2Rel"=11005, "ImicAxis_End"=11006, "ImicAxisXAbs"=11200, "ImicAxisYAbs"=11201, "ImicAxisZAbs"=11202, "ImicAxisTurretAbs"=11203, "ImicAxisFilter1Abs"=11204, "ImicAxisFilter2Abs"=11205, "ImicAxisXVel"=11300, "ImicAxisYVel"=11301, "ImicAxisZVel"=11302, "ImicAxisTurretVel"=11303, "ImicAxisFilter1Vel"=11304, "ImicAxisFilter2Vel"=11305, "ImicAxisXMoving"=11400, "ImicAxisYMoving"=11401, "ImicAxisZMoving"=11402, "ImicAxisTurretMoving"=11403, "ImicAxisFilter1Moving"=11404, "ImicAxisFilter2Moving"=11405, "ImicPiezoClip"=12001, "ImicPiezo"=12002, "IMIC_End"=12003] ("DeviceID")
                  # "LED:DA4:Range:0..5V\noder DO26=1025"
                  n69 = In Range and Coerce(upper limit=5.0 ("oberer Grenzwert"), x=w237, lower limit=-0.1 ("unterer Grenzwert")) -> (coerced(x)=w234:dbl)  [unwired: 1 out]
                  n70 = Bundle(cluster=w239, "Ring"=w238, "Value"=w234) -> (w240:cluster{"Ring":T3, "Value":dbl})
                }
                frame "led2" {
                  w241 = T3 1026 items=["EndLoop"=-2, "Loop"=-1, "Invalid"=0, "TriggerPolyV"=1, "TriggerCamera"=2, "SyncCamera"=3, "Do1"=1000, "Do2"=1001, "Do3"=1002, "Do4"=1003, "Do5"=1004, "Do6"=1005, "Do7"=1006, "Do8"=1007, "Do9"=1008, "Do10"=1009, "Do11"=1010, "Do12"=1011, "Do13"=1012, "Do14"=1013, "Do15"=1014, "Do16"=1015, "Do17"=1016, "Do18"=1017, "Do19"=1018, "Do20"=1019, "Do21"=1020, "Do22"=1021, "Do23"=1022, "Do24"=1023, "Do25"=1024, "Do26"=1025, "Do27"=1026, "Do28"=1027, "Do_End"=1028, "Da1"=2000, "Da2"=2001, "Da3"=2002, "Da4"=2003, "Da5"=2004, "Da6"=2005, "Da7"=2006, "Da8"=2007, "Da9"=2008, "Da10"=2009, "Da11"=2010, "Da12"=2011, "Da13"=2012, "Da14"=2013, "Da15"=2014, "Da16"=2015, "Da17"=2016, "Da18"=2017, "Da19"=2018, "DaLast"=2019, "Da1Incr"=2100, "Da2Incr"=2101, "Da3Incr"=2102, "Da4Incr"=2103, "Da5Incr"=2104, "Da6Incr"=2105, "Da7Incr"=2106, "Da8Incr"=2107, "Da1Raw"=2200, "Da2Raw"=2201, "Da3Raw"=2202, "Da4Raw"=2203, "Da5Raw"=2204, "Da6Raw"=2205, "Da7Raw"=2206, "Da8Raw"=2207, "Da1RawIncr"=2300, "Da2RawIncr"=2301, "Da3RawIncr"=2302, "Da4RawIncr"=2303, "Da5RawIncr"=2304, "Da6RawIncr"=2305, "Da7RawIncr"=2306, "Da8RawIncr"=2307, "Uart1"=3000, "Uart2"=3001, "Uart3"=3002, "Uart_End"=3003, "Di1"=4000, "Di2"=4001, "Di3"=4002, "Di4"=4003, "Di5"=4004, "Di6"=4005, "Di7"=4006, "Di8"=4007, "Di9"=4008, "Di10"=4009, "Di11"=4010, "Di12"=4011, "Di13"=4012, "Di14"=4013, "Di15"=4014, "Di16"=4015, "Di17"=4016, "Di18"=4017, "Di19"=4018, "Di20"=4019, "Di21"=4020, "Di22"=4021, "Di23"=4022, "Di24"=4023, "Di_End"=4024, "ICU_End"=4025, "LedIllum"=10000, "ImicAxisXRel"=11000, "ImicAxisYRel"=11001, "ImicAxisZRel"=11002, "ImicAxisTurretRel"=11003, "ImicAxisFilter1Rel"=11004, "ImicAxisFilter2Rel"=11005, "ImicAxis_End"=11006, "ImicAxisXAbs"=11200, "ImicAxisYAbs"=11201, "ImicAxisZAbs"=11202, "ImicAxisTurretAbs"=11203, "ImicAxisFilter1Abs"=11204, "ImicAxisFilter2Abs"=11205, "ImicAxisXVel"=11300, "ImicAxisYVel"=11301, "ImicAxisZVel"=11302, "ImicAxisTurretVel"=11303, "ImicAxisFilter1Vel"=11304, "ImicAxisFilter2Vel"=11305, "ImicAxisXMoving"=11400, "ImicAxisYMoving"=11401, "ImicAxisZMoving"=11402, "ImicAxisTurretMoving"=11403, "ImicAxisFilter1Moving"=11404, "ImicAxisFilter2Moving"=11405, "ImicPiezoClip"=12001, "ImicPiezo"=12002, "IMIC_End"=12003] ("Ring")
                  # "LED2 Range:0..5V\noder DO27=1026"
                  n71 = In Range and Coerce(upper limit=5.0 ("oberer Grenzwert"), x=w246, lower limit=-0.1 ("unterer Grenzwert")) -> (coerced(x)=w243:dbl)  [unwired: 1 out]
                  n72 = Bundle(cluster=w247, "Ring"=w241, "Value"=w243) -> (w248:cluster{"Ring":T3, "Value":dbl})
                }
                frame "led3" {
                  w249 = T3 1027 items=["EndLoop"=-2, "Loop"=-1, "Invalid"=0, "TriggerPolyV"=1, "TriggerCamera"=2, "SyncCamera"=3, "Do1"=1000, "Do2"=1001, "Do3"=1002, "Do4"=1003, "Do5"=1004, "Do6"=1005, "Do7"=1006, "Do8"=1007, "Do9"=1008, "Do10"=1009, "Do11"=1010, "Do12"=1011, "Do13"=1012, "Do14"=1013, "Do15"=1014, "Do16"=1015, "Do17"=1016, "Do18"=1017, "Do19"=1018, "Do20"=1019, "Do21"=1020, "Do22"=1021, "Do23"=1022, "Do24"=1023, "Do25"=1024, "Do26"=1025, "Do27"=1026, "Do28"=1027, "Do_End"=1028, "Da1"=2000, "Da2"=2001, "Da3"=2002, "Da4"=2003, "Da5"=2004, "Da6"=2005, "Da7"=2006, "Da8"=2007, "Da9"=2008, "Da10"=2009, "Da11"=2010, "Da12"=2011, "Da13"=2012, "Da14"=2013, "Da15"=2014, "Da16"=2015, "Da17"=2016, "Da18"=2017, "Da19"=2018, "DaLast"=2019, "Da1Incr"=2100, "Da2Incr"=2101, "Da3Incr"=2102, "Da4Incr"=2103, "Da5Incr"=2104, "Da6Incr"=2105, "Da7Incr"=2106, "Da8Incr"=2107, "Da1Raw"=2200, "Da2Raw"=2201, "Da3Raw"=2202, "Da4Raw"=2203, "Da5Raw"=2204, "Da6Raw"=2205, "Da7Raw"=2206, "Da8Raw"=2207, "Da1RawIncr"=2300, "Da2RawIncr"=2301, "Da3RawIncr"=2302, "Da4RawIncr"=2303, "Da5RawIncr"=2304, "Da6RawIncr"=2305, "Da7RawIncr"=2306, "Da8RawIncr"=2307, "Uart1"=3000, "Uart2"=3001, "Uart3"=3002, "Uart_End"=3003, "Di1"=4000, "Di2"=4001, "Di3"=4002, "Di4"=4003, "Di5"=4004, "Di6"=4005, "Di7"=4006, "Di8"=4007, "Di9"=4008, "Di10"=4009, "Di11"=4010, "Di12"=4011, "Di13"=4012, "Di14"=4013, "Di15"=4014, "Di16"=4015, "Di17"=4016, "Di18"=4017, "Di19"=4018, "Di20"=4019, "Di21"=4020, "Di22"=4021, "Di23"=4022, "Di24"=4023, "Di_End"=4024, "ICU_End"=4025, "LedIllum"=10000, "ImicAxisXRel"=11000, "ImicAxisYRel"=11001, "ImicAxisZRel"=11002, "ImicAxisTurretRel"=11003, "ImicAxisFilter1Rel"=11004, "ImicAxisFilter2Rel"=11005, "ImicAxis_End"=11006, "ImicAxisXAbs"=11200, "ImicAxisYAbs"=11201, "ImicAxisZAbs"=11202, "ImicAxisTurretAbs"=11203, "ImicAxisFilter1Abs"=11204, "ImicAxisFilter2Abs"=11205, "ImicAxisXVel"=11300, "ImicAxisYVel"=11301, "ImicAxisZVel"=11302, "ImicAxisTurretVel"=11303, "ImicAxisFilter1Vel"=11304, "ImicAxisFilter2Vel"=11305, "ImicAxisXMoving"=11400, "ImicAxisYMoving"=11401, "ImicAxisZMoving"=11402, "ImicAxisTurretMoving"=11403, "ImicAxisFilter1Moving"=11404, "ImicAxisFilter2Moving"=11405, "ImicPiezoClip"=12001, "ImicPiezo"=12002, "IMIC_End"=12003] ("Ring")
                  # "LED3:Range:0..5V\noder DO28=1027"
                  n73 = In Range and Coerce(upper limit=5.0 ("oberer Grenzwert"), x=w254, lower limit=-0.1 ("unterer Grenzwert")) -> (coerced(x)=w251:dbl)  [unwired: 1 out]
                  n74 = Bundle(cluster=w255, "Ring"=w249, "Value"=w251) -> (w256:cluster{"Ring":T3, "Value":dbl})
                }
                frame "led.intensity" {
                  w264 = 2016 items=["EndLoop"=-2, "Loop"=-1, "Invalid"=0, "TriggerPolyV"=1, "TriggerCamera"=2, "SyncCamera"=3, "Do1"=1000, "Do2"=1001, "Do3"=1002, "Do4"=1003, "Do5"=1004, "Do6"=1005, "Do7"=1006, "Do8"=1007, "Do9"=1008, "Do10"=1009, "Do11"=1010, "Do12"=1011, "Do13"=1012, "Do14"=1013, "Do15"=1014, "Do16"=1015, "Do17"=1016, "Do18"=1017, "Do19"=1018, "Do20"=1019, "Do21"=1020, "Do22"=1021, "Do23"=1022, "Do24"=1023, "Do_End"=1024, "Da1"=2000, "Da2"=2001, "Da3"=2002, "Da4"=2003, "Da5"=2004, "Da6"=2005, "Da7"=2006, "Da8"=2007, "Da17"=2016, "DaIncr_First"=2008, "Da1Incr"=2100, "Da2Incr"=2101, "Da3Incr"=2102, "Da4Incr"=2103, "Da5Incr"=2104, "Da6Incr"=2105, "Da7Incr"=2106, "Da8Incr"=2107, "Da1Raw"=2200, "Da2Raw"=2201, "Da3Raw"=2202, "Da4Raw"=2203, "Da5Raw"=2204, "Da6Raw"=2205, "Da7Raw"=2206, "Da8Raw"=2207, "Da1RawIncr"=2300, "Da2RawIncr"=2301, "Da3RawIncr"=2302, "Da4RawIncr"=2303, "Da5RawIncr"=2304, "Da6RawIncr"=2305, "Da7RawIncr"=2306, "Da8RawIncr"=2307, "Uart1"=3000, "Uart2"=3001, "Uart3"=3002, "Uart_End"=3003, "Di1"=4000, "Di2"=4001, "Di3"=4002, "Di4"=4003, "Di5"=4004, "Di6"=4005, "Di7"=4006, "Di8"=4007, "Di9"=4008, "Di10"=4009, "Di11"=4010, "Di12"=4011, "Di13"=4012, "Di14"=4013, "Di15"=4014, "Di16"=4015, "Di17"=4016, "Di18"=4017, "Di19"=4018, "Di20"=4019, "Di21"=4020, "Di22"=4021, "Di23"=4022, "Di24"=4023, "Di_End"=4024, "ICU_End"=4025, "LedIllum"=10000, "ImicAxisXRel"=11000, "ImicAxisYRel"=11001, "ImicAxisZRel"=11002, "ImicAxisTurretRel"=11003, "ImicAxisFilter1Rel"=11004, "ImicAxisFilter2Rel"=11005, "ImicAxis_End"=11006, "ImicAxisXAbs"=11200, "ImicAxisYAbs"=11201, "ImicAxisZAbs"=11202, "ImicAxisTurretAbs"=11203, "ImicAxisFilter1Abs"=11204, "ImicAxisFilter2Abs"=11205, "ImicAxisXVel"=11300, "ImicAxisYVel"=11301, "ImicAxisZVel"=11302, "ImicAxisTurretVel"=11303, "ImicAxisFilter1Vel"=11304, "ImicAxisFilter2Vel"=11305, "ImicAxisXMoving"=11400, "ImicAxisYMoving"=11401, "ImicAxisZMoving"=11402, "ImicAxisTurretMoving"=11403, "ImicAxisFilter1Moving"=11404, "ImicAxisFilter2Moving"=11405, "ImicPiezoClip"=12001, "ImicPiezo"=12002, "IMIC_End"=12003] ("DeviceID")
                  n75 = In Range and Coerce(upper limit=5.0 ("oberer Grenzwert"), x=w261, lower limit=0.0 ("unterer Grenzwert")) -> (coerced(x)=w260:dbl)  [unwired: 1 out]
                  n76 = Bundle(cluster=w258, "Ring"=w264, "Value"=w260) -> (w259:cluster{"Ring":T3, "Value":dbl})
                }
                frame "led2.intensity" {
                  w272 = 2017 items=["EndLoop"=-2, "Loop"=-1, "Invalid"=0, "TriggerPolyV"=1, "TriggerCamera"=2, "SyncCamera"=3, "Do1"=1000, "Do2"=1001, "Do3"=1002, "Do4"=1003, "Do5"=1004, "Do6"=1005, "Do7"=1006, "Do8"=1007, "Do9"=1008, "Do10"=1009, "Do11"=1010, "Do12"=1011, "Do13"=1012, "Do14"=1013, "Do15"=1014, "Do16"=1015, "Do17"=1016, "Do18"=1017, "Do19"=1018, "Do20"=1019, "Do21"=1020, "Do22"=1021, "Do23"=1022, "Do24"=1023, "Do_End"=1024, "Da1"=2000, "Da2"=2001, "Da3"=2002, "Da4"=2003, "Da5"=2004, "Da6"=2005, "Da7"=2006, "Da8"=2007, "Da17"=2016, "Da18"=2017, "Da19"=2018, "DaIncr_First"=2008, "Da1Incr"=2100, "Da2Incr"=2101, "Da3Incr"=2102, "Da4Incr"=2103, "Da5Incr"=2104, "Da6Incr"=2105, "Da7Incr"=2106, "Da8Incr"=2107, "Da1Raw"=2200, "Da2Raw"=2201, "Da3Raw"=2202, "Da4Raw"=2203, "Da5Raw"=2204, "Da6Raw"=2205, "Da7Raw"=2206, "Da8Raw"=2207, "Da1RawIncr"=2300, "Da2RawIncr"=2301, "Da3RawIncr"=2302, "Da4RawIncr"=2303, "Da5RawIncr"=2304, "Da6RawIncr"=2305, "Da7RawIncr"=2306, "Da8RawIncr"=2307, "Uart1"=3000, "Uart2"=3001, "Uart3"=3002, "Uart_End"=3003, "Di1"=4000, "Di2"=4001, "Di3"=4002, "Di4"=4003, "Di5"=4004, "Di6"=4005, "Di7"=4006, "Di8"=4007, "Di9"=4008, "Di10"=4009, "Di11"=4010, "Di12"=4011, "Di13"=4012, "Di14"=4013, "Di15"=4014, "Di16"=4015, "Di17"=4016, "Di18"=4017, "Di19"=4018, "Di20"=4019, "Di21"=4020, "Di22"=4021, "Di23"=4022, "Di24"=4023, "Di_End"=4024, "ICU_End"=4025, "LedIllum"=10000, "ImicAxisXRel"=11000, "ImicAxisYRel"=11001, "ImicAxisZRel"=11002, "ImicAxisTurretRel"=11003, "ImicAxisFilter1Rel"=11004, "ImicAxisFilter2Rel"=11005, "ImicAxis_End"=11006, "ImicAxisXAbs"=11200, "ImicAxisYAbs"=11201, "ImicAxisZAbs"=11202, "ImicAxisTurretAbs"=11203, "ImicAxisFilter1Abs"=11204, "ImicAxisFilter2Abs"=11205, "ImicAxisXVel"=11300, "ImicAxisYVel"=11301, "ImicAxisZVel"=11302, "ImicAxisTurretVel"=11303, "ImicAxisFilter1Vel"=11304, "ImicAxisFilter2Vel"=11305, "ImicAxisXMoving"=11400, "ImicAxisYMoving"=11401, "ImicAxisZMoving"=11402, "ImicAxisTurretMoving"=11403, "ImicAxisFilter1Moving"=11404, "ImicAxisFilter2Moving"=11405, "ImicPiezoClip"=12001, "ImicPiezo"=12002, "IMIC_End"=12003] ("DeviceID")
                  n77 = In Range and Coerce(upper limit=5.0 ("oberer Grenzwert"), x=w269, lower limit=0.0 ("unterer Grenzwert")) -> (coerced(x)=w268:dbl)  [unwired: 1 out]
                  n78 = Bundle(cluster=w266, "Ring"=w272, "Value"=w268) -> (w267:cluster{"Ring":T3, "Value":dbl})
                }
                frame "led3.intensity" {
                  w273 = T3 2018 items=["EndLoop"=-2, "Loop"=-1, "Invalid"=0, "TriggerPolyV"=1, "TriggerCamera"=2, "SyncCamera"=3, "Do1"=1000, "Do2"=1001, "Do3"=1002, "Do4"=1003, "Do5"=1004, "Do6"=1005, "Do7"=1006, "Do8"=1007, "Do9"=1008, "Do10"=1009, "Do11"=1010, "Do12"=1011, "Do13"=1012, "Do14"=1013, "Do15"=1014, "Do16"=1015, "Do17"=1016, "Do18"=1017, "Do19"=1018, "Do20"=1019, "Do21"=1020, "Do22"=1021, "Do23"=1022, "Do24"=1023, "Do25"=1024, "Do26"=1025, "Do27"=1026, "Do28"=1027, "Do_End"=1028, "Da1"=2000, "Da2"=2001, "Da3"=2002, "Da4"=2003, "Da5"=2004, "Da6"=2005, "Da7"=2006, "Da8"=2007, "Da9"=2008, "Da10"=2009, "Da11"=2010, "Da12"=2011, "Da13"=2012, "Da14"=2013, "Da15"=2014, "Da16"=2015, "Da17"=2016, "Da18"=2017, "Da19"=2018, "DaLast"=2019, "Da1Incr"=2100, "Da2Incr"=2101, "Da3Incr"=2102, "Da4Incr"=2103, "Da5Incr"=2104, "Da6Incr"=2105, "Da7Incr"=2106, "Da8Incr"=2107, "Da1Raw"=2200, "Da2Raw"=2201, "Da3Raw"=2202, "Da4Raw"=2203, "Da5Raw"=2204, "Da6Raw"=2205, "Da7Raw"=2206, "Da8Raw"=2207, "Da1RawIncr"=2300, "Da2RawIncr"=2301, "Da3RawIncr"=2302, "Da4RawIncr"=2303, "Da5RawIncr"=2304, "Da6RawIncr"=2305, "Da7RawIncr"=2306, "Da8RawIncr"=2307, "Uart1"=3000, "Uart2"=3001, "Uart3"=3002, "Uart_End"=3003, "Di1"=4000, "Di2"=4001, "Di3"=4002, "Di4"=4003, "Di5"=4004, "Di6"=4005, "Di7"=4006, "Di8"=4007, "Di9"=4008, "Di10"=4009, "Di11"=4010, "Di12"=4011, "Di13"=4012, "Di14"=4013, "Di15"=4014, "Di16"=4015, "Di17"=4016, "Di18"=4017, "Di19"=4018, "Di20"=4019, "Di21"=4020, "Di22"=4021, "Di23"=4022, "Di24"=4023, "Di_End"=4024, "ICU_End"=4025, "LedIllum"=10000, "ImicAxisXRel"=11000, "ImicAxisYRel"=11001, "ImicAxisZRel"=11002, "ImicAxisTurretRel"=11003, "ImicAxisFilter1Rel"=11004, "ImicAxisFilter2Rel"=11005, "ImicAxis_End"=11006, "ImicAxisXAbs"=11200, "ImicAxisYAbs"=11201, "ImicAxisZAbs"=11202, "ImicAxisTurretAbs"=11203, "ImicAxisFilter1Abs"=11204, "ImicAxisFilter2Abs"=11205, "ImicAxisXVel"=11300, "ImicAxisYVel"=11301, "ImicAxisZVel"=11302, "ImicAxisTurretVel"=11303, "ImicAxisFilter1Vel"=11304, "ImicAxisFilter2Vel"=11305, "ImicAxisXMoving"=11400, "ImicAxisYMoving"=11401, "ImicAxisZMoving"=11402, "ImicAxisTurretMoving"=11403, "ImicAxisFilter1Moving"=11404, "ImicAxisFilter2Moving"=11405, "ImicPiezoClip"=12001, "ImicPiezo"=12002, "IMIC_End"=12003] ("Ring")
                  n79 = In Range and Coerce(upper limit=5.0 ("oberer Grenzwert"), x=w278, lower limit=0.0 ("unterer Grenzwert")) -> (coerced(x)=w277:dbl)  [unwired: 1 out]
                  n80 = Bundle(cluster=w275, "Ring"=w273, "Value"=w277) -> (w276:cluster{"Ring":T3, "Value":dbl})
                }
              }
              n81 = case shown="No Error" w124 {
                selector: w124 -> [w287 w300]
                tunnel: [w286 w300] -> w127
                tunnel: w122 -> [w289 _]
                tunnel: w125 -> [w283 _]
                tunnel: w123 -> [w285 _]
                tunnel: w120 -> [w284 _]
                frame No Error {
                  n82 = Unbundle(w283) -> ("Ring"=w282:T3, "Value"=w281:dbl)
                  n83 = call "IMIC_SetDevice.vi"("Value"=w281, "DeviceID"=w282, "handle"=w289) -> ("output param"=w288:T4)  [unwired: 1 out]
                  n84 = case shown="\"no error\"" w288 {
                    selector: w288 -> [_ w297]
                    tunnel: w287 -> [w295 _]
                    tunnel: [w295 w299] -> w286
                    tunnel: w285 -> [w291 _]
                    tunnel: w284 -> [w290 _]
                    frame "no error" {
                      n85 = Number To Engineering String(1:FALSE ("use system decimal point (T)"), 4:w290) -> (0:w294:string)  [unwired: 2 out]
                      n86 = call "Variables.vi"("value"=w294, "Tag in"=w291, "Command"=T1."ChangeValue") -> ()  [unwired: 3 out]
                    }
                    frame "missing axis", Default {
                      # "sdk error"
                      n87 = Format Into String(w297) -> (resulting string=w296:string)  [unwired: 3 in, 1 out]
                      n88 = Bundle(TRUE, "output param"=w297, w296) -> (w299:T5)  [unwired: 1 out]
                    }
                  }
                }
                frame Error {
                }
              }
            }
          }
          "error out" <- w45
          n89 = call "ErrorLog.vi"("error in (no error)"=w45) -> ()  [unwired: 2 out]
        }
        n90 = Unbundle By Name(w39) -> ("status"=w43:bool)
      }
      n91 = call "IMIC_IsInit.vi"("handle"=w21) -> ("output param"=w22:T4, "handle out"=w20:u64)  [unwired: 1 out]
      n92 = case shown="\"no error\"" w22 {
        selector: w22 -> [_ w34]
        tunnel: [w33 w34] -> _
        tunnel: w20 -> [w32 _]
        frame "no error" {
          n93 = call "IMIC_Close.vi"("handle"=w32) -> ("output param"=w33:T4)  [unwired: 1 out]
        }
        frame "wrong handle", Default {
        }
      }
    }
    frame Error {
    }
  }
